vi "svl_Compute Frame and Perspective.vi"(0 "x scale":cluster{"x min":dbl, "x max":dbl} {"x max" format="%.2f"; "x min" format="%.2f"}, 1 "z scale":cluster{"z min":dbl, "z max":dbl} {"z max" format="%.2f"; "z min" format="%.2f"}, 2 "z axis height [%]":dbl format="%.2f", 3 "X maximum":dbl format="%.2f", 4 "Y maximum":dbl format="%.2f") -> (6 "front frame":cluster{dbl[], dbl[]} {"?" format="%.2f"; "?" format="%.2f"}, 7 "back frame":cluster{dbl[], dbl[]} {"?" format="%.2f"; "?" format="%.2f"}, 9 "dY":dbl format="%.2f", 10 "dX/dY":dbl format="%.2f")   [LabVIEW 2017]
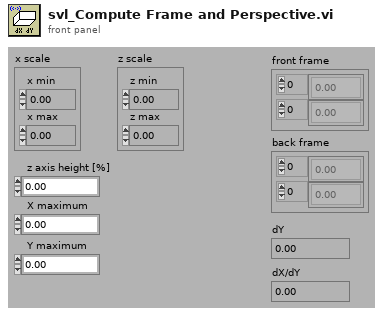
[diagram p1: front panel]
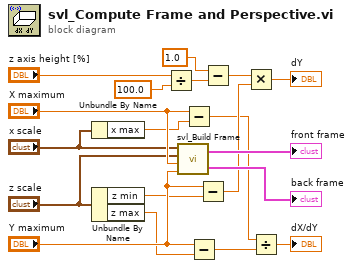
[diagram p0: block diagram]
diagram:
  n1 = Unbundle By Name("x scale") -> ("x max"=w1:dbl)
  n2 = Unbundle By Name("z scale") -> ("z min"=w4:dbl, "z max"=w3:dbl)
  n3 = Divide(x="z axis height [%]", y=100.0) -> (x/y=w11:dbl)
  n4 = call <vilib>:"svl_Build Frame.vi"("Y maximum"="Y maximum", "X maximum"="X maximum", "z scale"="z scale", "x scale"="x scale") -> ("back frame"=→"back frame":cluster{dbl[], dbl[]}, "front frame"=→"front frame":cluster{dbl[], dbl[]})
  n5 = Subtract(x="X maximum", y=w1) -> (x-y=w8:dbl)
  n6 = Subtract(x="Y maximum", y=w3) -> (x-y=w7:dbl)
  n7 = Subtract(x="Y maximum", y=w4) -> (x-y=w15:dbl)
  n8 = Subtract(x=1.0, y=w11) -> (x-y=w14:dbl)
  n9 = Multiply(x=w14, y=w15) -> (x*y=→"dY":dbl)
  n10 = Divide(x=w8, y=w7) -> (x/y=→"dX/dY":dbl)
